vi "Actor Core.vi"(8 "error in":errorcluster, 11 "MFC Actor.lvlib:MFC.lvclass":refnum<class "MFC.lvclass">) -> (0 "error out":errorcluster, 3 "Actor out":refnum<class "Actor.lvclass">)   [LabVIEW 2013, in "MFC.LVLIB" / "MFC.lvclass"]
doc: "This is Actor Core.vi, the main message handling loop for Actors. An actor usually just sits in this loop and processes messages as they arrive. Any error returned by the message Do.vi call will stop the loop, with error code 43 as the canonical signal to stop with no error sent to caller. Descendants may override that in Handle Error.vi."
uses:
  MFC.lvclass
  PluginInterface/Actor Framework.lvlibp/Actor/Actor.lvclass
  MFC.lvclass/MFC.ctl
  PluginInterface/PluginInterface.lvlibp/PluginInterfaceClass/PluginInterface.lvclass
  PluginInterface/Actor Framework.lvlibp/Message Enqueuer/Message Priority.ctl
  Write Graph.vi
  Write Setpoint.vi
  Write Value.vi
  Write Graph History.vi
  PluginInterface/PluginInterface.lvlibp/PluginInterfaceClass/Write VI Refnum.vi
  PluginInterface/Actor Framework.lvlibp/Message Enqueuer/Enqueue.vi
  MFC Messages/Initialize Msg/Initialize Msg.lvclass
  MFC Messages/Update Graphs Msg/Update Graphs Msg.lvclass
  MFC Messages/Update Setpoint Msg/Update Setpoint Msg.lvclass
  MFC Messages/Write MFC Msg/Write MFC Msg.lvclass
  MFC Messages/Read MFC Msg/Read MFC Msg.lvclass
  MFC Messages/Log Data Msg/Log Data Msg.lvclass
  PluginInterface/Actor Framework.lvlibp/Stop Msg/Stop Msg.lvclass
  PluginInterface/Actor Framework.lvlibp/Message Enqueuer/Message Enqueuer.lvclass
panel:
  in  "stop signal":bool
  in  "Round Color Box 4":u32(colorbox)=16728642
  in  "Round Color Box 3":u32(colorbox)=483491
  in  "Setpoint 1":dbl=36.41913854673561
  out "Value 1":dbl=36.53012927910604
  in  "Graph History":dbl=300.0
  out "Graph 1":T1(graph)
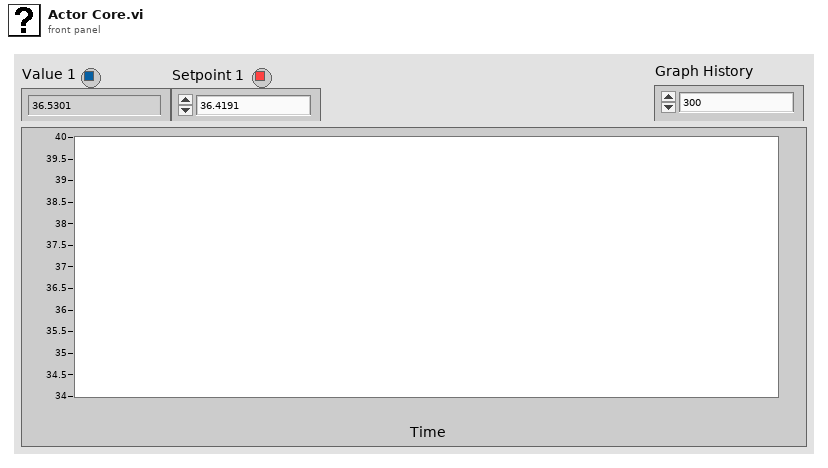
[diagram p1: front panel]
types:
  T1 = cluster{"output array":dbl[], "output array":dbl[]}[]
  T2 = typedef "Actor Framework.lvlibp/Message Enqueuer.lvclass/Message Priority.ctl" = enum16{"Low", "Normal", "High"}
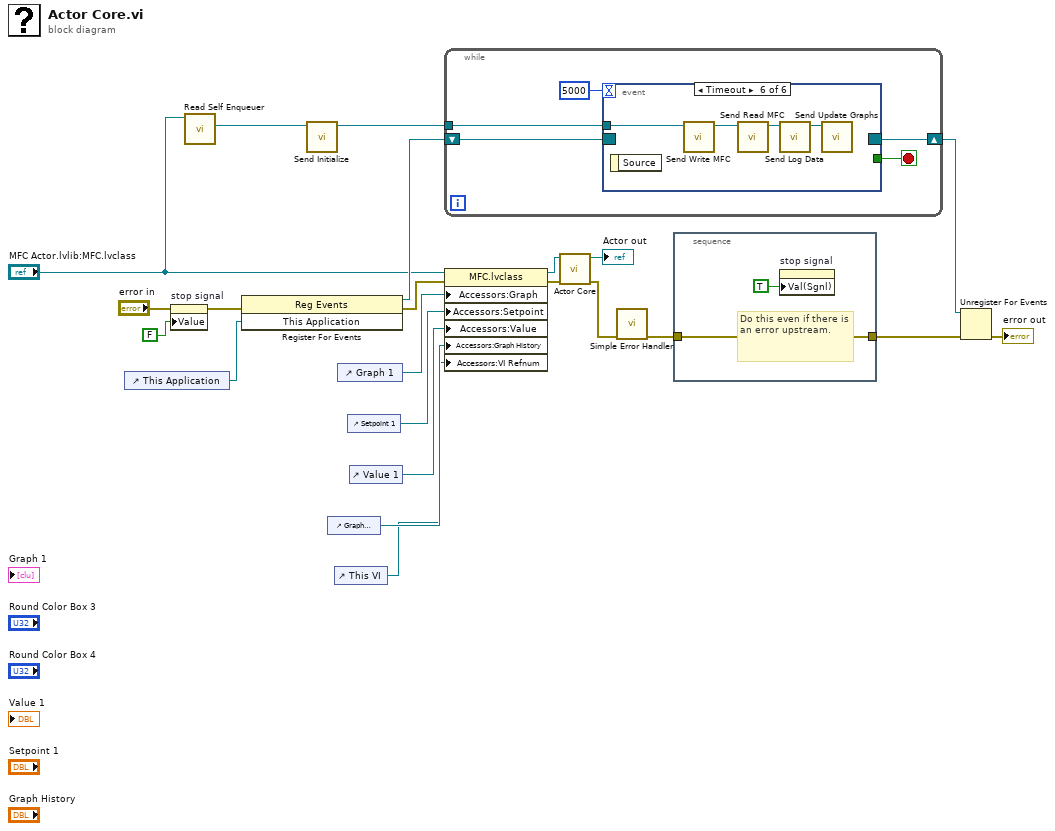
[diagram p0: block diagram]
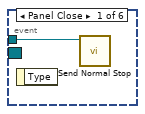
[diagram p2: hidden frame]
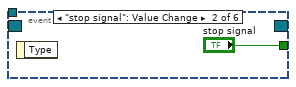
[diagram p3: hidden frame]
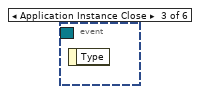
[diagram p4: hidden frame]
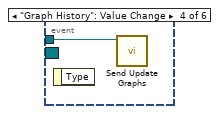
[diagram p5: hidden frame]
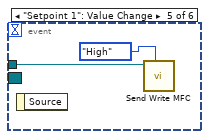
[diagram p6: hidden frame]
diagram:
  n1 = control-ref of="This Application"() -> (w15:refnum<vi>)
  n2 = property on="stop signal" class="Bool (strict)"(error in="error in", "Value"=FALSE ("stop")) -> (error out=w16:errorcluster)  [unwired: 1 in, 1 out]
  n3 = call "Read Self Enqueuer.vi"("Actor"="MFC Actor.lvlib:MFC.lvclass") -> ("Self Enqueuer"=w4:refnum<class "Message Enqueuer.lvclass">)  [unwired: 10 in]
  n4 = register-events(error in=w16, w15) -> (reference out=w19:refnum<event-registration>, error out=w2:errorcluster)  [unwired: 1 in]
  n5 = call "Send Initialize.vi"("Message Enqueuer"=w4) -> ("Message Enqueuer out"=w3:refnum<class "Message Enqueuer.lvclass">)  [unwired: 9 in, 1 out]
  n6 = control-ref of="Graph History"() -> (w6:refnum<vi>)
  n7 = control-ref of="This VI"() -> (w1:refnum<vi>)
  n8 = control-ref of="Graph 1"() -> (w5:refnum<vi>)
  n9 = control-ref of="Setpoint 1"() -> (w8:refnum<vi>)
  n10 = control-ref of="Value 1"() -> (w9:refnum<vi>)
  n11 = while {
    tunnel: w3 -> [w27]
    shift-right: [w24] -> w18
    shift-left: w19 -> [w25]
    stop <- w26 stop-if-true
    n12 = event shown="[5] Timeout" {
      selector: w25 -> [_ _ _ _ _ _]
      dyn-events: [_ _ _ _ _ _] -> w24
      timeout: 5000 -> [_ _ _ _ _ _]
      tunnel: w27 -> [w28 _ _ w30 w32 w36]
      tunnel: [_ "stop signal" _ _ _ _] -> w26
      event Panel Close {
        n13 = event-data() -> ()  [unwired: 1 in, 1 out]
        n14 = call "Send Normal Stop.vi"("Message Enqueuer"=w28) -> ()  [unwired: 10 in, 1 out]
      }
      event "stop signal": Value Change {
        n15 = event-data() -> ()  [unwired: 1 in, 1 out]
      }
      event Application Instance Close {
        n16 = event-data() -> ()  [unwired: 1 in, 1 out]
      }
      event "Graph History": Value Change {
        n17 = event-data() -> ()  [unwired: 1 in, 1 out]
        n18 = call "Send Update Graphs.vi"("Message Enqueuer"=w30) -> ()  [unwired: 9 in, 2 out]
      }
      event "Setpoint 1": Value Change {
        n19 = event-data() -> ()  [unwired: 1 in, 1 out]
        n20 = call "Send Write MFC.vi"("Message Priority (Normal)"=Message_Priority."High", "Message Enqueuer"=w32) -> ()  [unwired: 8 in, 2 out]
      }
      event Timeout {
        n21 = event-data() -> ()  [unwired: 1 in, 1 out]
        n22 = call "Send Write MFC.vi"("Message Enqueuer"=w36) -> ("Message Enqueuer out"=w33:refnum<class "Message Enqueuer.lvclass">)  [unwired: 9 in, 1 out]
        n23 = call "Send Read MFC.vi"("Message Enqueuer"=w33) -> ("Message Enqueuer out"=w35:refnum<class "Message Enqueuer.lvclass">)  [unwired: 9 in, 1 out]
        n24 = call "Send Log Data.vi"("Message Enqueuer"=w35) -> ("Message Enqueuer out"=w34:refnum<class "Message Enqueuer.lvclass">)  [unwired: 9 in, 1 out]
        n25 = call "Send Update Graphs.vi"("Message Enqueuer"=w34) -> ()  [unwired: 9 in, 2 out]
      }
    }
  }
  n26 = property class="MFC.lvclass"(reference="MFC Actor.lvlib:MFC.lvclass", error in=w2, "Accessors:Graph"=w5, "Accessors:Setpoint"=w8, "Accessors:Value"=w9, "Accessors:Graph History"=w6, "Accessors:VI Refnum"=w1) -> (reference out=w14:refnum<class "MFC.lvclass">, error out=w10:errorcluster)
  n27 = call-parent "Actor Core.vi"("error in"=w10, "Actor in"=w14) -> ("error out"=w21:errorcluster, "Actor out"=→"Actor out":refnum<class "Actor.lvclass">)  [unwired: 8 in]
  n28 = call <vilib>:"Simple Error Handler.vi"("error in (no error)"=w21) -> ("error out"=w20:errorcluster)  [unwired: 4 in, 4 out]
  n29 = stacked-sequence {
    tunnel: [w37] -> w17
    tunnel: w20 -> [w37]
    frame #0 {
      # "Do this even if there is an error upstream."
      n30 = property on="stop signal" class="Bool (strict)"("Val(Sgnl)"=TRUE ("stop")) -> ()  [unwired: 2 in, 2 out]
    }
  }
  n31 = Unregister For Events(event registration refnum=w18, error in=w17) -> (error out=→"error out":errorcluster)
